vi "anonymous_cluster_identity.vi"(11 "cluster_in":cluster{"first":dbl, "second":dbl}) -> (3 "cluster_out":cluster{"first":dbl, "second":dbl})   [LabVIEW 2020]
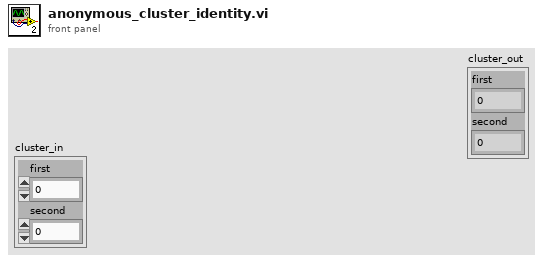
[diagram p1: front panel]
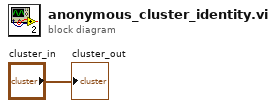
[diagram p0: block diagram]
diagram:
  "cluster_out" <- "cluster_in"
